vi "基础19.vi"() -> ()   [LabVIEW 2014]
panel:
  out "数值 2":dbl
  out "数值":dbl
  in  "停止":bool
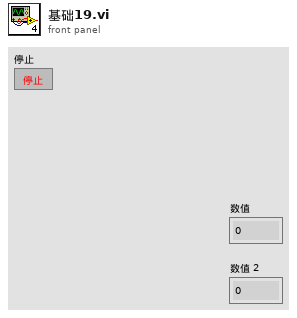
[diagram p1: front panel]
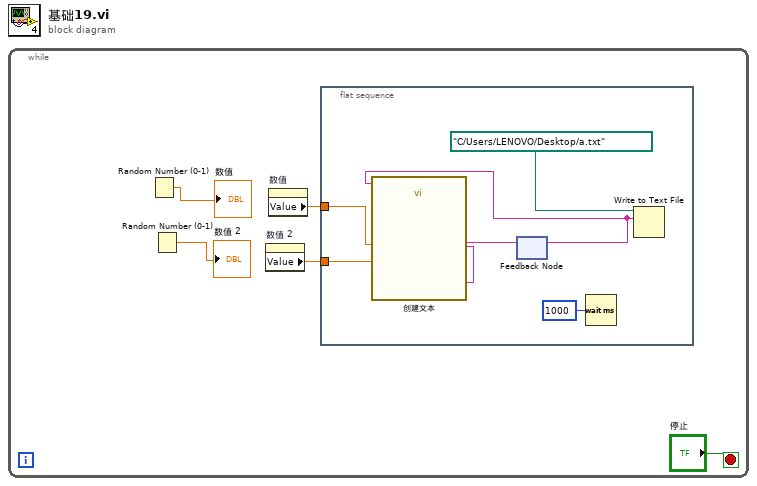
[diagram p0: block diagram]
diagram:
  n1 = while {
    stop <- "停止" stop-if-true
    n2 = Random Number (0-1)() -> (number: 0 to 1=→"数值":dbl)
    n3 = Random Number (0-1)() -> (number: 0 to 1=→"数值 2":dbl)
    n4 = property on="数值 2" class="DigNum (严格)"() -> ("Value"=w1:dbl)  [unwired: 2 in, 2 out]
    n5 = property on="数值" class="DigNum (严格)"() -> ("Value"=w2:dbl)  [unwired: 2 in, 2 out]
    n6 = flat-sequence {
      tunnel: w2 -> [w11]
      tunnel: w1 -> [w10]
      frame #0 {
        n7 = feedback #1() -> (w6:string)  [unwired: 1 in]
        n8 = call "创建文本"("Beginning Text"=w6, "n"=w11, "m"=w10) -> ("Result"=w7:string)  [unwired: 11 in, 1 out]
        n9 = feedback-in #1(w7) -> ()
        n10 = Wait (ms)(milliseconds to wait=u32 1000 ("等待时间（毫秒）")) -> ()  [unwired: 1 out]
        n11 = Write to Text File(file (use dialog)=path "C:/Users/LENOVO/Desktop/a.txt" ("文件（使用对话框）"), text=w6) -> ()  [unwired: 2 in, 3 out]
      }
    }
  }
